vi "Show exe.vi"(8 "error in (no error)":errorcluster, 10 "Show":enum16{"False", "True"}(ring), 11 "LT_UpgradeFlash in":refnum<class "LT_UpgradeFlash.lvclass">) -> (0 "error out":errorcluster, 3 "LT_UpgradeFlash out":refnum<class "LT_UpgradeFlash.lvclass">)   [LabVIEW 2017, in "LT_UpgradeFlash.lvclass"]
uses:
  LT_UpgradeFlash.lvclass
  D:/Project/Tymphany/LT_UpgradeFlash/New_Lib/LT_UpgradeFlash_dll/LT_UpgradeFlash_dll/bin/Debug/LT_UpgradeFlash_dll.dll
  New_Lib/LT_UpgradeFlash_dll/LT_UpgradeFlash_dll/bin/Debug/LT_UpgradeFlash_dll.dll
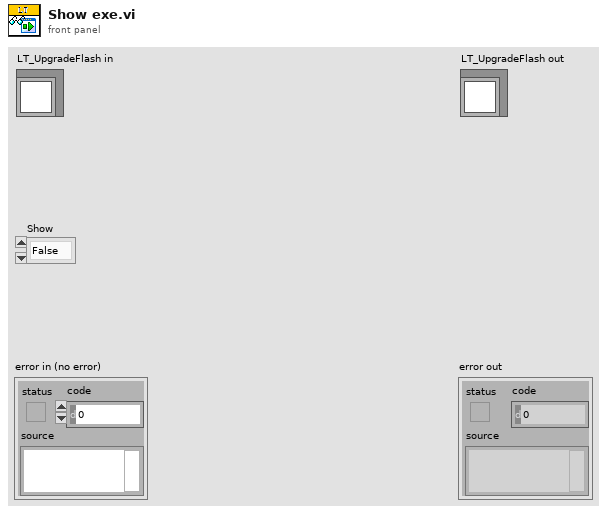
[diagram p1: front panel]
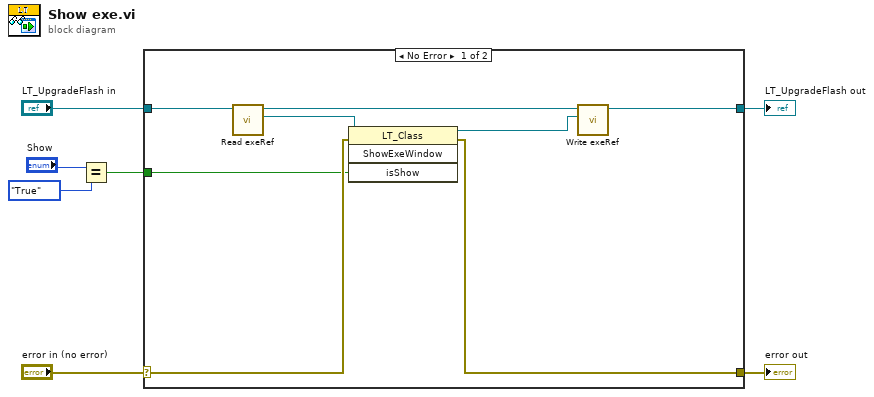
[diagram p0: block diagram]
diagram:
  n1 = Equal?(x="Show", y=enum16{"False", "True"}."True") -> (x = y?=w1:bool)
  n2 = case shown="No Error" "error in (no error)" {
    selector: "error in (no error)" -> [w13 w17]
    tunnel: [w12 w17] -> w6
    tunnel: [w9 w16] -> w4
    tunnel: "LT_UpgradeFlash in" -> [w15 w16]
    tunnel: w1 -> [w8 _]
    frame No Error {
      n3 = call-dynamic "Read exeRef.vi"("LT_UpgradeFlash in"=w15) -> ("exeRef"=w14:refnum<k24>, "LT_UpgradeFlash out"=w10:refnum<class "LT_UpgradeFlash.lvclass">)  [unwired: 8 in, 1 out]
      n4 = invoke class="LT_Class" method="ShowExeWindow"(reference=w14, error in=w13, "isShow"=w8) -> (reference out=w11:refnum<k24>, error out=w12:errorcluster)  [unwired: 1 in, 2 out]
      n5 = call-dynamic "Write exeRef.vi"("exeRef"=w11, "LT_UpgradeFlash in"=w10) -> ("LT_UpgradeFlash out"=w9:refnum<class "LT_UpgradeFlash.lvclass">)  [unwired: 8 in, 1 out]
    }
    frame Error {
    }
  }
  "error out" <- w6
  "LT_UpgradeFlash out" <- w4
